vi "testGetPropertyFromAddedConfigurationFileWithoutDeploying.vi"(8 "error in (no error)":errorcluster, 11 "TestCase in":refnum<class "VeriStandTestCaseUnitTests.lvclass">) -> (0 "error out":errorcluster, 3 "TestCase out":refnum<class "VeriStandTestCaseUnitTests.lvclass">)   [LabVIEW 2027, in "VeriStandTestCaseUnitTests.lvclass"]
uses:
  VeriStandTestCaseUnitTests.lvclass
  Source/VeriStandTestCase/VeriStandTestCase.lvclass
  <vilib>/addons/_JKI Toolkits/VI Tester/TestCase.llb/TestCase.lvclass
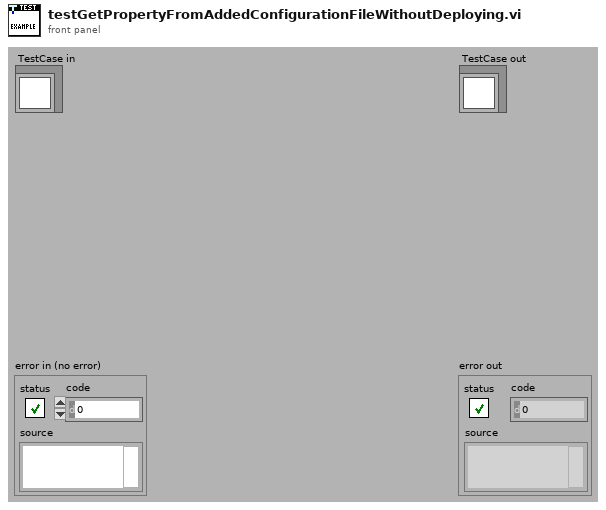
[diagram p1: front panel]
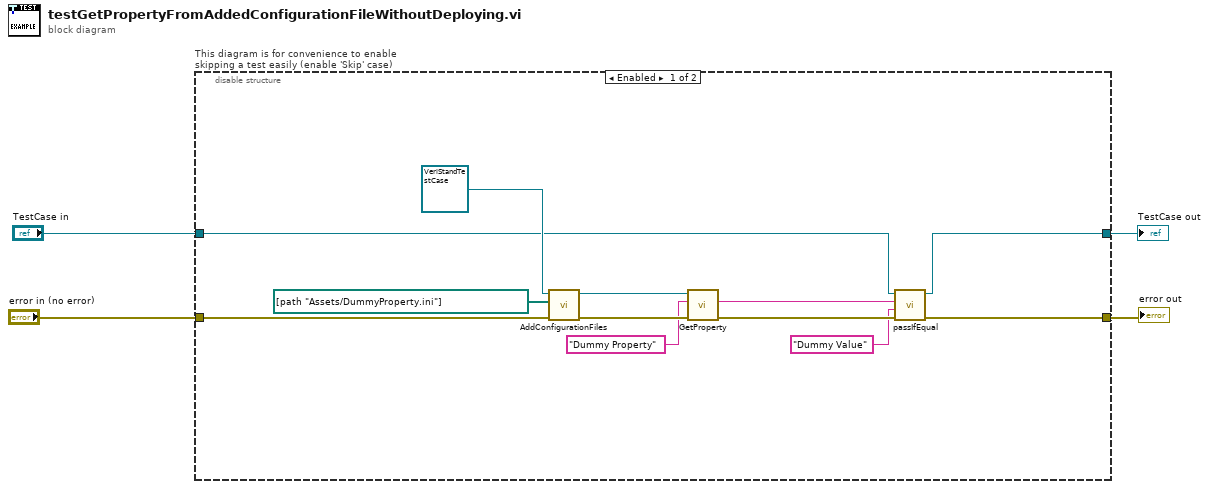
[diagram p0: block diagram]
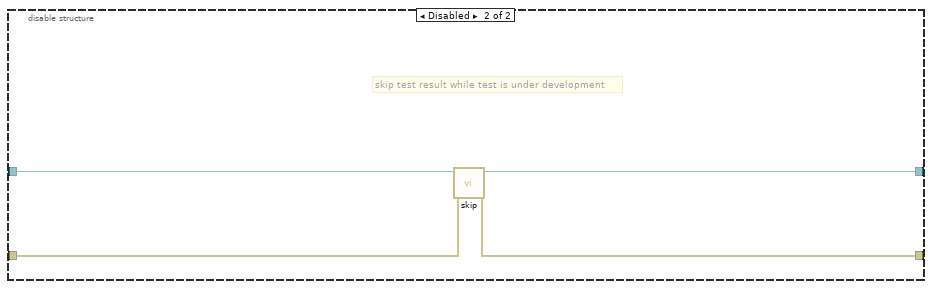
[diagram p2: hidden frame]
diagram:
  n1 = disable-structure "This diagram is for convenience to enable skipping a test easily (enable 'Skip' case)" shown="Enabled" {
    disable-tunnel: "TestCase in" -> [w8 w20]
    disable-tunnel: [w7 w18] -> w1
    disable-tunnel: [w9 w19] -> w3
    disable-tunnel: "error in (no error)" -> [w16 w17]
    frame Enabled {
      n2 = call "AddConfigurationFiles.vi"("error in (no error)"=w16, "configuration files"=path[] [path "Assets/DummyProperty.ini"], "VeriStandTestCase in"=refnum<class "VeriStandTestCase.lvclass"> refnum ("VeriStand Test Case in")) -> ("error out"=w13:errorcluster, "VeriStandTestCase out"=w11:refnum<class "VeriStandTestCase.lvclass">)  [unwired: 7 in]
      n3 = call "GetProperty.vi"("error in (no error)"=w13, "key"="Dummy Property", "VeriStandTestCase in"=w11) -> ("error out"=w12:errorcluster, "value"=w6:string)  [unwired: 6 in, 1 out]
      n4 = call-dynamic "passIfEqual.vi"("error in (no error)"=w12, "y"="Dummy Value" ("key"), "x"=w6, "TestCase in"=w8) -> ("error out"=w9:errorcluster, "TestCase out"=w7:refnum<class "VeriStandTestCaseUnitTests.lvclass">)  [unwired: 6 in]
    }
    frame Disabled {
      # "skip test result while test is under development"
      n5 = call <vilib>:"skip.vi"("error in (no error)"=w17, "TestCase in"=w20) -> ("error out"=w19:errorcluster, "TestCase out"=w18:refnum<class "VeriStandTestCaseUnitTests.lvclass">)  [unwired: 8 in]
    }
  }
  "error out" <- w3
  "TestCase out" <- w1
